vi "TEST_Direct Cmds.vi"() -> ()   [LabVIEW 2012]
panel:
  out "voltage":dbl(knob) scale=-10.0..10.0
  out "Btns":T1
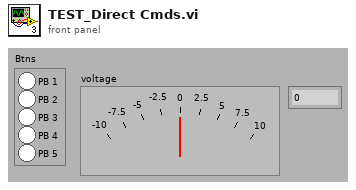
[diagram p1: front panel]
types:
  T1 = cluster{"PB 1":bool, "PB 2":bool, "PB 3":bool, "PB 4":bool, "PB 5":bool}
  T2 = typedef "BotSpeak_Control.ctl" = cluster{"Address":string, "Reply EOF":string, "Hardware":path, "Retries":i8, "Timeout":i32}
  T3 = cluster{"[0]":bool, "[1]":bool, "[2]":bool, "[3]":bool, "[4]":bool}
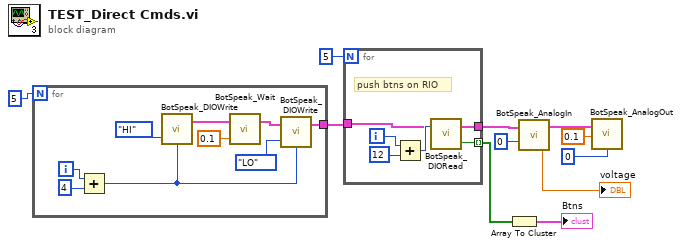
[diagram p0: block diagram]
diagram:
  n1 = for {
    N: 5 -> [_]
    tunnel: [w12] -> w1
    i -> [w20]
    n2 = Add(x=w20, y=4) -> (x+y=w14:i32)
    n3 = call <userlib>:"BotSpeak_DIOWrite.vi"("State"=enum32{"LO", "HI"}."HI", "DIO Line"=w14) -> ("Bot Settings"=w16:T2)  [unwired: 1 in, 1 out]
    n4 = call <userlib>:"BotSpeak_Wait.vi"("Wait (sec)"=0.1, "Bot Settings"=w16) -> ("Bot Settings"=w15:T2)  [unwired: 1 in]
    n5 = call <userlib>:"BotSpeak_DIOWrite.vi"("State"=enum32{"LO", "HI"}."LO", "Bot Settings"=w15, "DIO Line"=w14) -> ("Bot Settings"=w12:T2)  [unwired: 1 out]
  }
  n6 = for {
    N: 5 -> [_]
    tunnel: w1 -> [w23]
    tunnel: [w21] -> w9 mode=indexing
    tunnel: [w22] -> w6
    i -> [w25]
    # "push btns on RIO"
    n7 = Add(x=w25, y=12) -> (x+y=w24:i32)
    n8 = call <userlib>:"BotSpeak_DIORead.vi"("Bot Settings"=w23, "DIO Line"=w24) -> ("State"=w21:bool, "Bot Settings out"=w22:T2)  [unwired: 1 in]
  }
  n9 = Array To Cluster(array=w9) -> (cluster=→"Btns":T3)
  n10 = call <userlib>:"BotSpeak_AnalogIn.vi"("Bot Settings"=w6, "A/D Channel"=u8 0) -> ("voltage"=→"voltage":dbl, "Bot Settings"=w3:T2)  [unwired: 1 in]
  n11 = call <userlib>:"BotSpeak_AnalogOut.vi"("voltage"=0.1, "Bot Settings"=w3, "DAC Channel"=u8 0) -> ()  [unwired: 2 out]
